vi "BRig_RT_comm_webdav_upload_all_warnUser.vi"(9 "input_n":i32, 10 "input_arrFilenames":string[](array[string]), 11 "input_arrUploaded":bool[](array[boolean])) -> ()   [LabVIEW 2014]
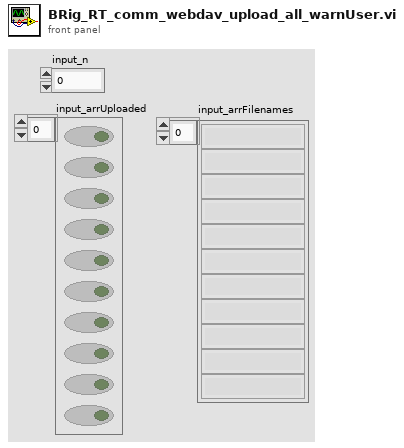
[diagram p1: front panel]
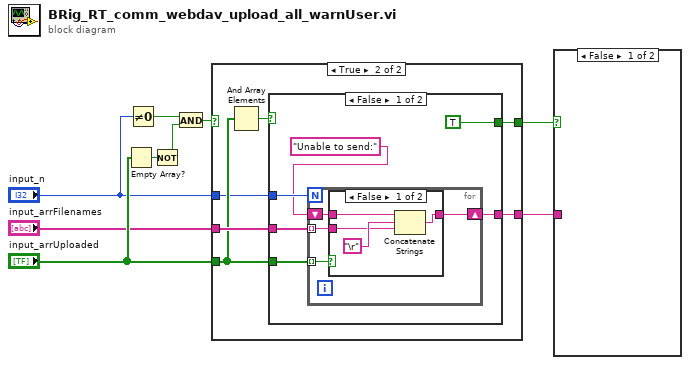
[diagram p0: block diagram]
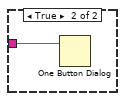
[diagram p2: hidden frame]
diagram:
  n1 = Empty Array?(array="input_arrUploaded") -> (empty?=w9:bool)
  n2 = Not Equal To 0?(x="input_n") -> (x != 0?=w8:bool)
  n3 = Not(x=w9) -> (.not. x?=w7:bool)
  n4 = And(x=w8, y=w7) -> (x .and. y?=w6:bool)
  n5 = case shown="True" w6 {
    tunnel: "input_arrUploaded" -> [_ w13]
    tunnel: "input_arrFilenames" -> [_ w14]
    tunnel: "input_n" -> [_ w12]
    tunnel: [_ w11] -> w1
    tunnel: [_ w10] -> w2
    frame False {
    }
    frame True {
      n6 = And Array Elements(Boolean array=w13) -> (logical AND=w15:bool)
      n7 = case shown="False" w15 {
        tunnel: w14 -> [w20 _]
        tunnel: w13 -> [w19 _]
        tunnel: w12 -> [w21 _]
        tunnel: [w18 _] -> w11
        tunnel: [TRUE _] -> w10
        frame False {
          n8 = for {
            N: w21 -> [_]
            tunnel: w20 -> [w23] mode=indexing
            tunnel: w19 -> [w25] mode=indexing
            shift-right: [w22] -> w18
            shift-left: "Unable to send:" -> [w24]
            n9 = case shown="False" w25 {
              tunnel: w24 -> [w29 w30]
              tunnel: [w28 w30] -> w22
              tunnel: w23 -> [w26 _]
              frame False {
                n10 = Concatenate Strings(w29, "\r", w26) -> (w28:string)
              }
              frame True {
              }
            }
          }
        }
        frame True {
        }
      }
    }
  }
  n11 = case shown="False" w2 {
    tunnel: w1 -> [_ w31]
    frame False {
    }
    frame True {
      n12 = One Button Dialog(message=w31) -> ()  [unwired: 1 in, 1 out]
    }
  }
